vi "sub_UDP_Listener.vi"(8 "error in (no error)":errorcluster, 11 "UDP Network Connection in":refnum<k16>) -> (0 "error out":errorcluster, 2 "Packets":string[](array[string]), 3 "Received Packet":bool=TRUE)   [LabVIEW 2012]
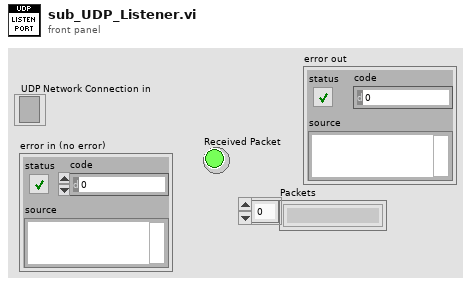
[diagram p1: front panel]
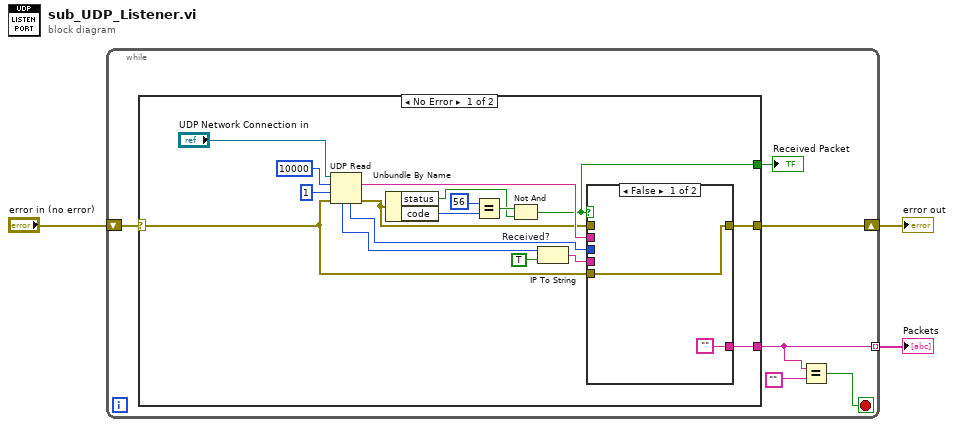
[diagram p0: block diagram]
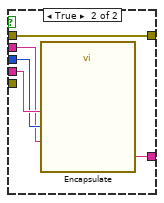
[diagram p2: hidden frame]
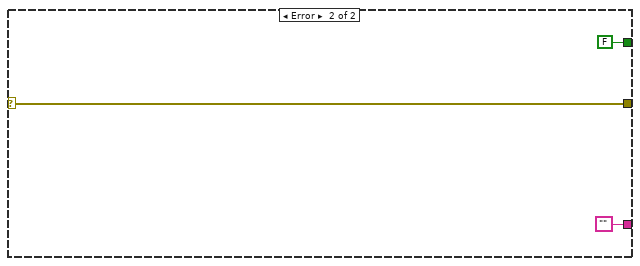
[diagram p3: hidden frame]
diagram:
  n1 = while {
    tunnel: [w6] -> w3 mode=indexing
    shift-right: [w8] -> w2
    shift-left: "error in (no error)" -> [w7]
    stop <- w4 stop-if-true
    n2 = case shown="No Error" w7 {
      selector: w7 -> [w10 w34]
      tunnel: [w22 ""] -> w6
      tunnel: [w15 FALSE] -> w9
      tunnel: [w12 w34] -> w8
      frame No Error {
        n3 = UDP Read(connection ID="UDP Network Connection in", max size (548)=10000, timeout ms (25000)=1, 8:w10) -> (data out=w23:string, error out=w11:errorcluster, 4:w18:u16, 6:w21:u32)  [unwired: 1 out]
        n4 = Unbundle By Name(w11) -> ("status"=w13:bool, "code"=w16:i32)
        n5 = Equal?(x=56 ("y"), y=w16) -> (x = y?=w14:bool)
        n6 = Not And "Received?"(1:w13, 2:w14) -> (0:w15:bool)
        n7 = IP To String(1:TRUE ("dot notation? (F)"), 2:w21) -> (0:w19:string)
        n8 = case shown="False" w15 {
          tunnel: w23 -> [_ w30]
          tunnel: ["" w32] -> w22
          tunnel: w19 -> [_ w33]
          tunnel: w18 -> [_ w31]
          tunnel: [w27 w29] -> w12
          tunnel: w10 -> [w27 _]
          tunnel: w11 -> [_ w29]
          frame False {
          }
          frame True {
            n9 = call "Encapsulate"("src.ip"=w33, "src.port"=w31, "Packet Content"=w30) -> ("Result"=w32:string)  [unwired: 11 in, 1 out]
          }
        }
      }
      frame Error {
      }
    }
    "Received Packet" <- w9
    n10 = Equal?(x=w6, y="") -> (x = y?=w4:bool)
  }
  "Packets" <- w3
  "error out" <- w2
